vi "PH_AxisGUI_BaseClass.ProcCases.vi"(0 "i ref in":refnum<vi>, 1 "selector":string, 2 "data":i8[](array[numeric]), 3 "call cluster":T1={"Object"="", "Selector"="", "CallType"=enum."synchronous", "Async Object"="", "Async Selector"="", "Data Descriptor"="", "Data"=[], "Error #"=0, "Expire"=0}, 5 "error in":errorcluster) -> (14 "i ref out":refnum<vi>, 17 "answer cluster":T1={"Object"="", "Selector"="", "CallType"=enum."synchronous", "Async Object"="", "Async Selector"="", "Data Descriptor"="", "Data"=[], "Error #"=0, "Expire"=0}, 19 "error out":errorcluster)   [LabVIEW 2014, in "PH_AxisGUI_BaseClass.lvlib"]
doc: "This method is called by a process from within the default case in the event loop. The methods of a class that are linked to events will be called from THIS method. Add your code here."
uses:
  PH_AxisGUI_BaseClass.lvlib
  CS_Core/CSSystem/CoreDefs/CoreDefs.call_type.ctl
  CS_Core/BaseProcess/BaseProcess.descriptor string definition.ctl
  CS_Core/CSSystem/CoreDefs/CoreDefs.rawDataType.ctl
  CS_Core/CSSystem/CoreLib/CoreLib.string 2 byte array.vi
  CS_Core/BaseProcess/BaseProcess.lvlib
  CS_Core/CSSystem/CoreLib/CoreLib.lvlib
  CS_Core/CAEObj/CAEObj.lvlib
  PH_Stepmotor_BaseClass/PH_Stepmotor_BaseClass.lvlib
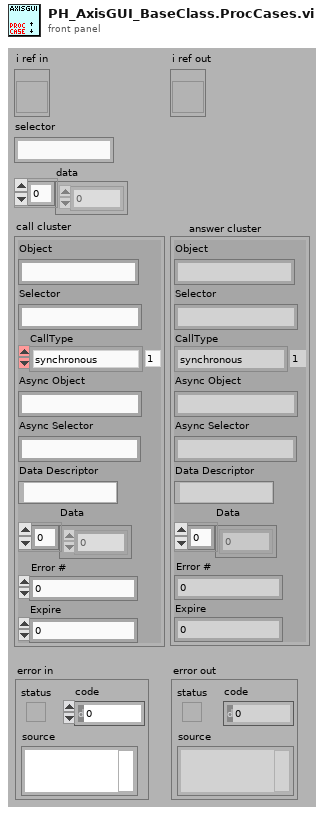
[diagram p1: front panel]
types:
  T1 = typedef "CoreDefs.call_type.ctl" = cluster{"Object":string, "Selector":string, "CallType":enum16{"simple", "synchronous", "asynchronous"}, "Async Object":string, "Async Selector":string, "Data Descriptor":T2, "Data":T3, "Error #":i32, "Expire":u32}
  T2 = typedef "BaseProcess.lvlib/BaseProcess.descriptor string definition.ctl" = string
  T3 = typedef "CoreDefs.rawDataType.ctl" = i8[]
  T4 = typedef "PH_Stepmotor_BaseClass.lvlib/PH_Stepmotor_BaseClass.Axis Settings.ctl" = cluster{"Sign change":bool, "Width":dbl, "Calibration":dbl, "Unit":string, "Motor Type":T5, "Unit Width":string, "Unit CF":string}
  T5 = typedef "PH_Stepmotor_BaseClass.lvlib/PH_Stepmotor_BaseClass.Motor Type.ctl" = enum16{"Unspecific", "OWIS 49.120.2633", "OWIS 49.060.1033", "OWIS 43.040.2558", "Diamond Motion 2200 series", "OWIS 49.120.266B.MV6", "Calorimeter", "Linear Stage 1", "MICOS VT-80", "MICOS VT-80 S", "Standa Rotstage nt0.95A", "PUF RA 320.200", "PUF RA 800.200", "PUF RA 800.400", "PUF RA 400.50", "1324.nn.800.50", "1324.n9c.800.50", "1324.nn.320.200", "1324.nn.400.200", "1324.nn.800.200", "1324.nn.400.50", "1324.8c9c.800.50", "1324.8c9c.400.200"}
  T6 = typedef "PH_Stepmotor_BaseClass.lvlib/PH_Stepmotor_BaseClass.Axis Information.ctl" = cluster{"Scaled Position":dbl, "Activity":T7}
  T7 = typedef "PH_Stepmotor_BaseClass.lvlib/PH_Stepmotor_BaseClass.Axis Activity.ctl" = enum16{"No Information", "stopped", "running", "Failure", "Alarm", "stopped at backward ES", "stopped at foreward ES"}
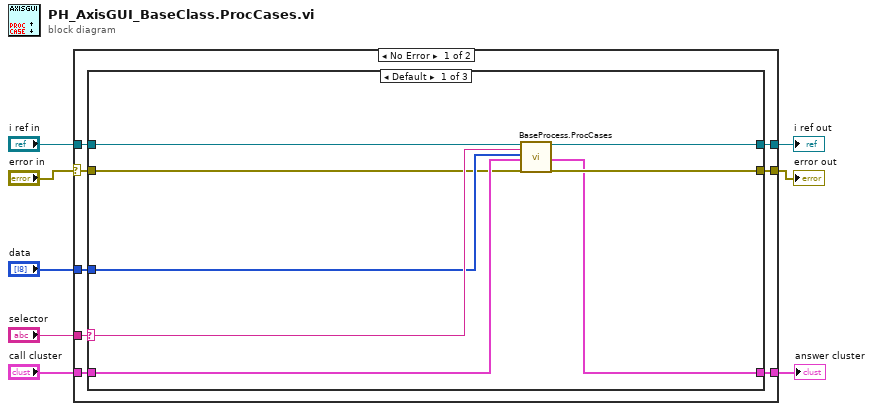
[diagram p0: block diagram]
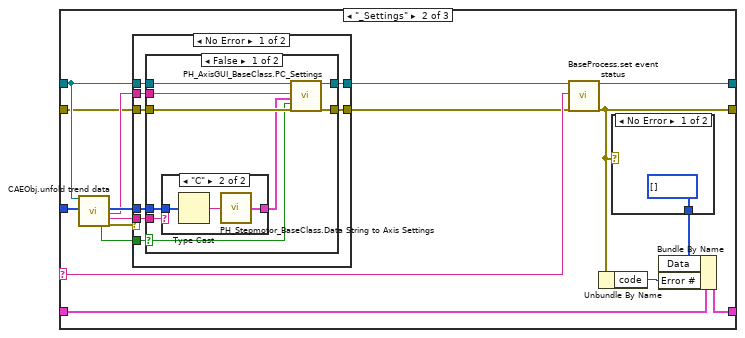
[diagram p2: hidden frame]
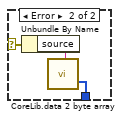
[diagram p6: hidden frame]
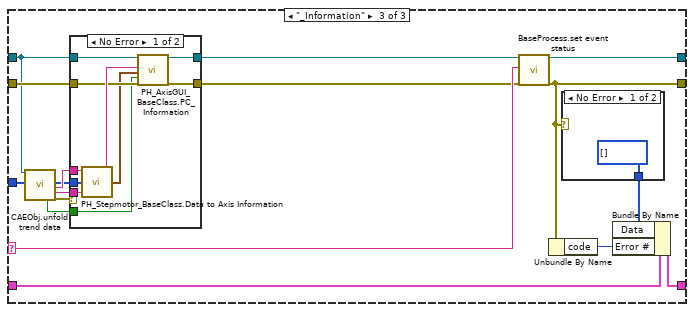
[diagram p7: hidden frame]
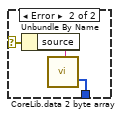
[diagram p9: hidden frame]
diagram:
  n1 = case shown="No Error" "error in" {
    selector: "error in" -> [w9 w103]
    tunnel: "selector" -> [w16 _]
    tunnel: [w15 w102] -> w7
    tunnel: "call cluster" -> [w14 w102]
    tunnel: "i ref in" -> [w13 w104]
    tunnel: [w12 w104] -> w4
    tunnel: [w11 w103] -> w3
    tunnel: "data" -> [w10 _]
    frame No Error {
      n2 = case shown="Default" w16 {
        selector: w16 -> [w20 w35 w83]
        tunnel: w13 -> [w19 w29 w70]
        tunnel: [w24 w38 w82] -> w12
        tunnel: w14 -> [w21 w40 w85]
        tunnel: [w22 w36 w80] -> w15
        tunnel: w9 -> [w17 w28 w74]
        tunnel: [w23 w39 w84] -> w11
        tunnel: w10 -> [w18 w27 w71]
        frame Default {
          n3 = call "BaseProcess.ProcCases.vi"("i ref in"=w19, "selector"=w20, "Data"=w18, "call cluster"=w21, "error in (no error)"=w17) -> ("i ref out"=w24:refnum<vi>, "answer cluster"=w22:T1, "error out"=w23:errorcluster)  [unwired: 12 in]
        }
        frame "_Settings" {
          n4 = call "CAEObj.unfold trend data.vi"("i ref in"=w29, "raw trend data"=w27) -> ("no link"=w34:bool, "data"=w31:i8[], "serviceName"=w30:string, "typeDescriptor"=w33:string, "error out"=w32:errorcluster)  [unwired: 9 in, 4 out]
          n5 = case shown="No Error" w32 {
            tunnel: w31 -> [w44 _]
            tunnel: w29 -> [w48 w65]
            tunnel: [w47 w65] -> w26
            tunnel: w28 -> [w49 w64]
            tunnel: [w46 w64] -> w25
            tunnel: w34 -> [w45 _]
            tunnel: w33 -> [w43 _]
            tunnel: w30 -> [w42 _]
            frame No Error {
              n6 = case "NO LINK?" shown="False" w45 {
                selector: w45 -> [w50 _]
                tunnel: w49 -> [w57 w63]
                tunnel: w48 -> [w58 w62]
                tunnel: [w54 w62] -> w47
                tunnel: [w53 w63] -> w46
                tunnel: w43 -> [w55 _]
                tunnel: w44 -> [w56 _]
                tunnel: w42 -> [w52 _]
                frame False {
                  n7 = case shown="\"C\"" w55 {
                    tunnel: [_ w59] -> w51
                    tunnel: w56 -> [_ w61]
                    frame Default {
                    }
                    frame "C" {
                      n8 = Type Cast(x=w61) -> (*(type *) &x=w60:string)  [unwired: 1 in]
                      n9 = call "PH_Stepmotor_BaseClass.Data String to Axis Settings.vi"("Data String"=w60) -> ("Axis Settings"=w59:T4)  [unwired: 1 out]
                    }
                  }
                  n10 = call "PH_AxisGUI_BaseClass.PC_Settings.vi"("i ref in"=w58, "Service Name"=w52, "Axis Settings"=w51, "No Link?"=w50, "error in"=w57) -> ("i ref out"=w54:refnum<vi>, "error"=w53:errorcluster)  [unwired: 12 in, 1 out]
                }
                frame True {
                }
              }
            }
            frame Error {
            }
          }
          n11 = call "BaseProcess.set event status.vi"("i ref in"=w26, "EventStatus"=w35, "error in (no error)"=w25) -> ("i ref out"=w38:refnum<vi>, "error out"=w39:errorcluster)  [unwired: 14 in, 1 out]
          n12 = Unbundle By Name(w39) -> ("code"=w41:i32)
          n13 = case shown="No Error" w39 {
            selector: w39 -> [_ w69]
            tunnel: [T3 [] ("byteArray out") w67] -> w37
            frame No Error {
            }
            frame Error {
              n14 = Unbundle By Name(w69) -> ("source"=w68:string)
              n15 = call-poly "CoreLib.data 2 byte array.vi"("string"=w68) -> ("byteArray out"=w67:T3)  [unwired: 18 in]
            }
          }
          n16 = Bundle By Name(cluster=w40, "Data"=w37, "Error #"=w41) -> (w36:T1)
        }
        frame "_Information" {
          n17 = call "CAEObj.unfold trend data.vi"("i ref in"=w70, "raw trend data"=w71) -> ("no link"=w75:bool, "data"=w78:i8[], "serviceName"=w79:string, "typeDescriptor"=w76:string, "error out"=w77:errorcluster)  [unwired: 9 in, 4 out]
          n18 = case shown="No Error" w77 {
            tunnel: w78 -> [w94 _]
            tunnel: w70 -> [w92 w97]
            tunnel: [w88 w97] -> w72
            tunnel: w74 -> [w91 w96]
            tunnel: w75 -> [w89 _]
            tunnel: w76 -> [w93 _]
            tunnel: w79 -> [w95 _]
            tunnel: [w87 w96] -> w73
            frame No Error {
              n19 = call "PH_Stepmotor_BaseClass.Data to Axis Information.vi"("data"=w94, "Type Descriptor"=w93) -> ("Axis Information"=w90:T6)
              n20 = call "PH_AxisGUI_BaseClass.PC_Information.vi"("i ref in"=w92, "Service Name"=w95, "Axis Information"=w90, "no link"=w89, "error in"=w91) -> ("i ref out"=w88:refnum<vi>, "error out"=w87:errorcluster)  [unwired: 12 in, 1 out]
            }
            frame Error {
            }
          }
          n21 = call "BaseProcess.set event status.vi"("i ref in"=w72, "EventStatus"=w83, "error in (no error)"=w73) -> ("i ref out"=w82:refnum<vi>, "error out"=w84:errorcluster)  [unwired: 14 in, 1 out]
          n22 = Unbundle By Name(w84) -> ("code"=w86:i32)
          n23 = case shown="No Error" w84 {
            selector: w84 -> [_ w101]
            tunnel: [T3 [] ("byteArray out") w99] -> w81
            frame No Error {
            }
            frame Error {
              n24 = Unbundle By Name(w101) -> ("source"=w100:string)
              n25 = call-poly "CoreLib.data 2 byte array.vi"("string"=w100) -> ("byteArray out"=w99:T3)  [unwired: 18 in]
            }
          }
          n26 = Bundle By Name(cluster=w85, "Data"=w81, "Error #"=w86) -> (w80:T1)
        }
      }
    }
    frame Error {
    }
  }
  "answer cluster" <- w7
  "i ref out" <- w4
  "error out" <- w3
